vi "Port2-5 Serial Driver Start.vi"() -> (0 "driver opened":bool[](array[boolean]))   [LabVIEW 2024]
uses:
  Globals and TypeDefs/SerpOpen.vi
panel:
  in  "input driver names":string[](array[string])=[".aIn", ".bIn", ".cIn", ".dIn", ".eIn", ".fIn"]
  in  "out driver names":string[](array[string])=[".aOut", ".bOut", ".cOut", ".dOut", ".eOut", ".fOut"]
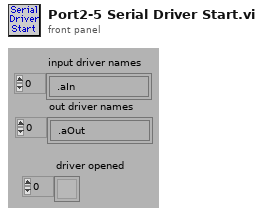
[diagram p1: front panel]
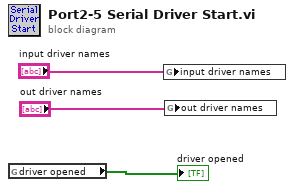
[diagram p0: block diagram]
diagram:
  n1 = global read "SerpOpen.vi" "driver opened"() -> (→"driver opened":bool[])
  n2 = global write "SerpOpen.vi" "input driver names"("input driver names") -> ()
  n3 = global write "SerpOpen.vi" "out driver names"("out driver names") -> ()
